vi "Send Message.vi"(5 "Target Task":u32, 7 "Target Node":u32, 8 "error in (no error)":errorcluster, 9 "Type ID":u32, 10 "Payload":u8[](array[numeric]), 11 "TCPMessageService in":refnum<class "TCPMessageAPI.lvclass">) -> (0 "error out":errorcluster, 3 "TCPMessageService out":refnum<class "TCPMessageAPI.lvclass">)   [LabVIEW 2020, in "Vecto.lvlib" / "TCPMessageAPI.lvclass"]
uses:
  TCPMessageAPI.lvclass
  proto/TcpPayload/Data.ctl
  TCPMessageAPI.lvclass/TCPMessageAPI.ctl
  proto/TcpPayload/TcpPayload.lvlib
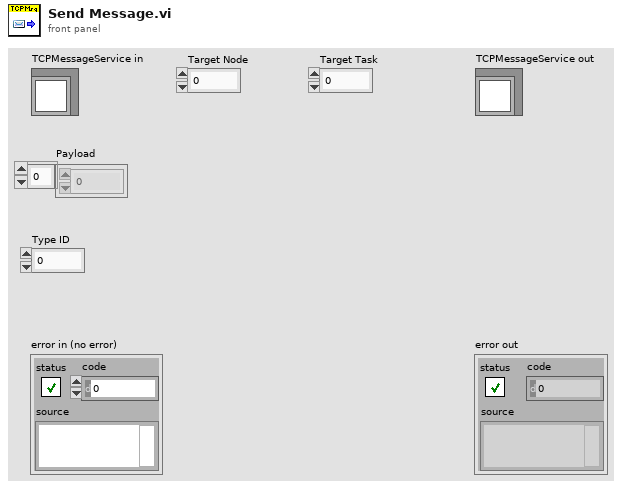
[diagram p1: front panel]
types:
  T1 = typedef "TcpPayload.lvlib/Data.ctl" = cluster{"target_node":u32, "target_task":u32, "source_id":u32, "sequence":u32, "timestamp":u64, "type_id":u32, "payload":u8[]}
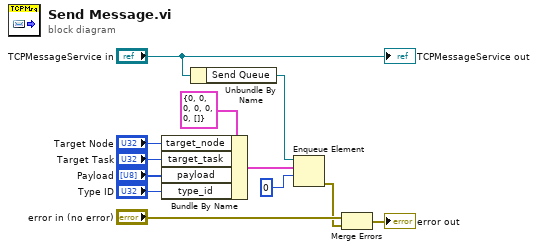
[diagram p0: block diagram]
diagram:
  n1 = Bundle By Name(cluster=T1 {"target_node"=0, "target_task"=0, "source_id"=0, "sequence"=0, "timestamp"=0, "type_id"=0, "payload"=[]} ("TcpPayload"), "target_node"="Target Node", "target_task"="Target Task", "payload"="Payload", "type_id"="Type ID") -> (w1:T1)
  n2 = Unbundle By Name("TCPMessageService in") -> ("Send Queue"=w6:refnum<queue>)
  n3 = Enqueue Element(queue=w6, element=w1, timeout in ms (-1)=0) -> (error out=w2:errorcluster)  [unwired: 1 in, 2 out]
  n4 = Merge Errors("error in (no error)", w2) -> (→"error out":errorcluster)
  "TCPMessageService out" <- "TCPMessageService in"
